vi "ARN Test Aktiv.vi"(11 "error in (no error)":errorcluster caption="Fehler (Eingang, kein Fehler)", 13 "Aktion":T1(ring)) -> (4 "ARN Test Aktiv":bool, 15 "error out":errorcluster caption="Fehler (Ausgang)")   [LabVIEW 2020, in "EPA 1065.lvlib" / "ARN Test 1065-305.lvlib"]
uses:
  ARN Test 1065-305.lvlib
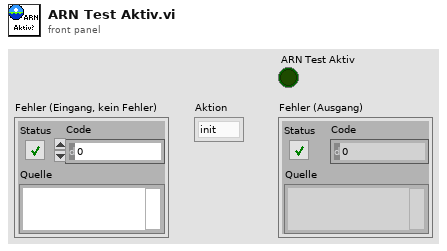
[diagram p1: front panel]
types:
  T1 = enum16{"init", "lesen", "ARN Test aktiv", "ARN Test inaktiv"}
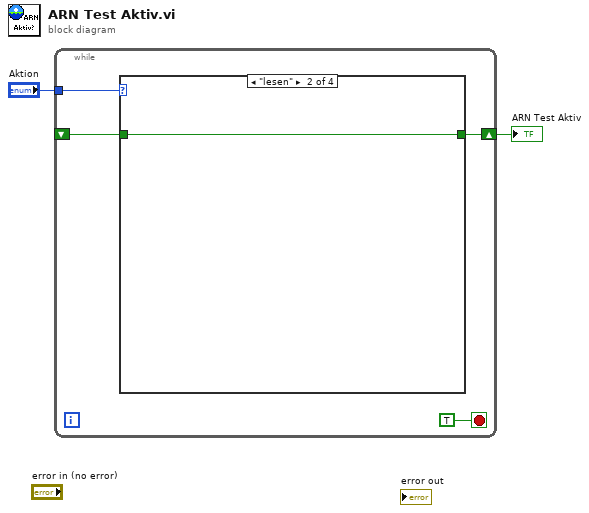
[diagram p0: block diagram]
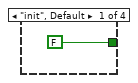
[diagram p2: hidden frame]
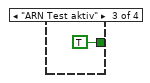
[diagram p3: hidden frame]
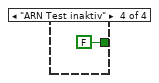
[diagram p4: hidden frame]
diagram:
  n1 = while {
    tunnel: "Aktion" -> [w5]
    shift-right: [w4] -> w1
    shift-left: _ -> [w3]
    stop <- TRUE stop-if-true
    n2 = case shown="\"lesen\"" w5 {
      tunnel: [FALSE w8 TRUE FALSE] -> w4
      tunnel: w3 -> [_ w8 _ _]
      frame "init", Default {
      }
      frame "lesen" {
      }
      frame "ARN Test aktiv" {
      }
      frame "ARN Test inaktiv" {
      }
    }
  }
  "ARN Test Aktiv" <- w1
